vi "Kr_rel_corr_2024.vi"(0 "N2 rel freq / Hz":dbl, 1 "O2 rel freq / Hz":dbl, 2 "Frequency / Hz":dbl, 3 "N2 rel strength":dbl, 4 "O2 rel strength":dbl) -> (5 "Kr":dbl)   [LabVIEW 2016]
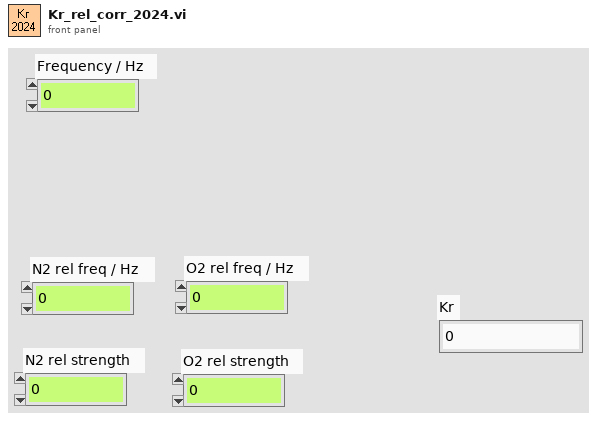
[diagram p1: front panel]
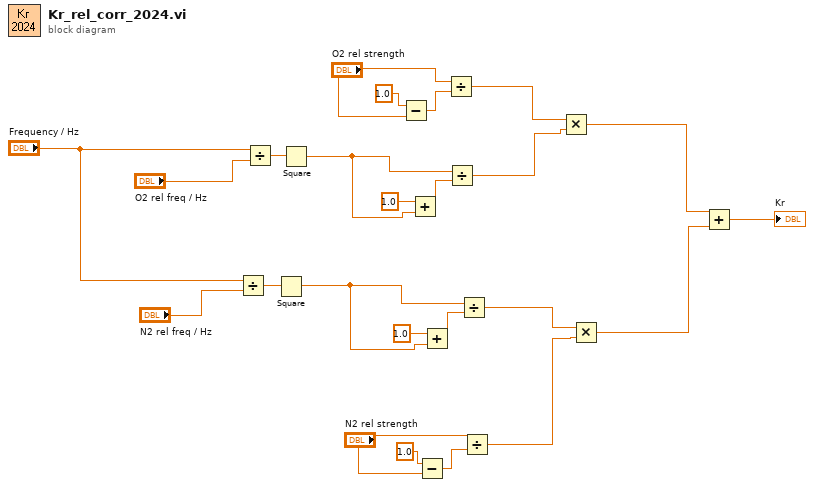
[diagram p0: block diagram]
diagram:
  n1 = Divide(x="Frequency / Hz", y="N2 rel freq / Hz") -> (x/y=w14:dbl)
  n2 = Divide(x="Frequency / Hz", y="O2 rel freq / Hz") -> (x/y=w15:dbl)
  n3 = Square(x=w14) -> (x^2=w8:dbl)
  n4 = Square(x=w15) -> (x^2=w11:dbl)
  n5 = Subtract(x=1.0, y="O2 rel strength") -> (x-y=w24:dbl)
  n6 = Add(x=1.0, y=w11) -> (x+y=w13:dbl)
  n7 = Subtract(x=1.0, y="N2 rel strength") -> (x-y=w21:dbl)
  n8 = Add(x=1.0, y=w8) -> (x+y=w10:dbl)
  n9 = Divide(x="O2 rel strength", y=w24) -> (x/y=w7:dbl)
  n10 = Divide(x=w11, y=w13) -> (x/y=w6:dbl)
  n11 = Divide(x=w8, y=w10) -> (x/y=w5:dbl)
  n12 = Divide(x="N2 rel strength", y=w21) -> (x/y=w4:dbl)
  n13 = Multiply(x=w7, y=w6) -> (x*y=w3:dbl)
  n14 = Multiply(x=w5, y=w4) -> (x*y=w2:dbl)
  n15 = Add(x=w3, y=w2) -> (x+y=→"Kr":dbl)
